vi "WPI_DashboardNT Log FieldName Cache.vi"(9 "Index":i32, 10 "Name":string, 11 "Operation":enum16{"Lookup/Add", "Index", "Clear"}(ring)=enum."Clear") -> (0 "New/Valid":bool, 1 "Index out":i32, 2 "Name out":string)   [LabVIEW 2017]
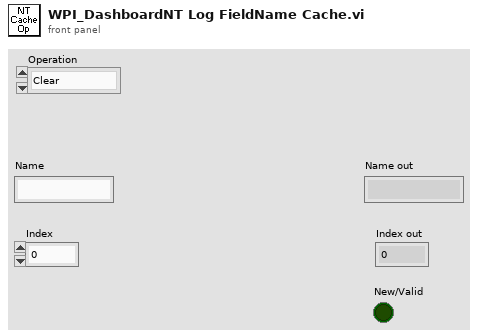
[diagram p1: front panel]
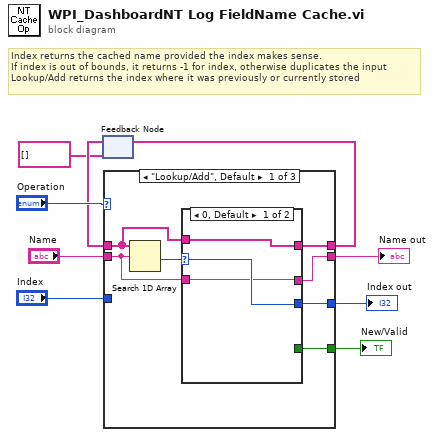
[diagram p0: block diagram]
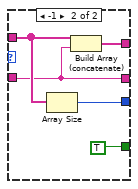
[diagram p2: hidden frame]
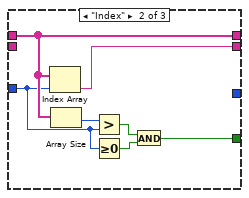
[diagram p3: hidden frame]
diagram:
  # "Index returns the cached name provided the index makes sense.\nIf index is out of bounds, it returns -1 for index, otherwise duplicates the input\nLookup/Add returns the index where it was previously or currently stored"
  n1 = feedback #1(string[] []) -> (w5:string[])
  n2 = case shown="\"Lookup/Add\", Default" "Operation" {
    tunnel: "Index" -> [_ w28 w32]
    tunnel: [w10 w31 _] -> w7
    tunnel: "Name" -> [w14 _ _]
    tunnel: w5 -> [w15 w30 _]
    tunnel: [w13 w30 _] -> w3
    tunnel: [w12 _ w32] -> w2
    tunnel: [w11 w25 _] -> w1
    frame "Lookup/Add", Default {
      n3 = Search 1D Array(1D array=w15, element=w14) -> (index of element=w16:i32)  [unwired: 1 in]
      n4 = case shown="0, Default" w16 {
        selector: w16 -> [w19 _]
        tunnel: w15 -> [w18 w23]
        tunnel: w14 -> [w17 w20]
        tunnel: [w18 w24] -> w13
        tunnel: [w19 w22] -> w12
        tunnel: [_ TRUE] -> w11
        tunnel: [w17 w20] -> w10
        frame 0, Default {
        }
        frame -1 {
          n5 = Array Size(array=w23) -> (size(s)=w22:i32)
          n6 = Build Array (concatenate)(w23, w20) -> (w24:string[])
        }
      }
    }
    frame "Index" {
      n7 = Index Array(array=w30, index=w28) -> (element=w31:string)
      n8 = Array Size(array=w30) -> (size(s)=w29:i32)
      n9 = Greater?(x=w29, y=w28) -> (0:w27:bool)
      n10 = Greater Or Equal To 0?(x=w28) -> (x >= 0?=w26:bool)
      n11 = And(x=w27, y=w26) -> (x .and. y?=w25:bool)
    }
    frame "Clear" {
    }
  }
  "Name out" <- w7
  "Index out" <- w2
  "New/Valid" <- w1
  n12 = feedback-in #1(w3) -> ()
